vi "UICtrls_BuildMessage.vi"(1 "Control Label":string, 2 "Control Data":variant) -> (7 "Data":variant)   [LabVIEW 2025, in "UI_Library.lvlib"]
doc: "Build Message for UI Handler Loop"
uses:
  UI_Library.lvlib
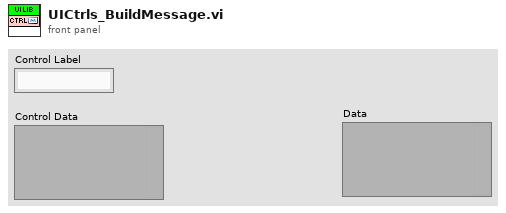
[diagram p1: front panel]
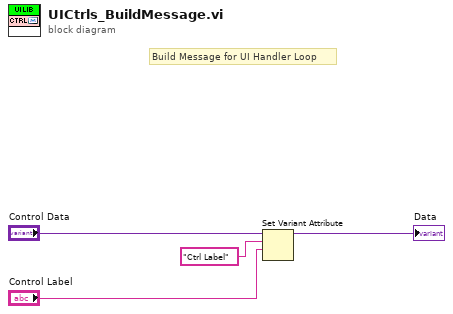
[diagram p0: block diagram]
diagram:
  # "Build Message for UI Handler Loop"
  n1 = Set Variant Attribute(Variant="Control Data", name="Ctrl Label" ("Control Label"), value="Control Label") -> (Variant out=→"Data":variant)  [unwired: 1 in, 2 out]
